vi "Parse XML.vi"(10 "Sender Host":string, 11 "Message XML String":string) -> (3 "Message":T2)   [LabVIEW 2014, in "AMC.lvlib"]
uses:
  AMC.lvlib
  Keyed Array/KeyedArray.ctl
  Keyed Array/Tools_KeyedArray.lvlib
  TypeDefs/Message.ctl
panel:
  out "Attributes":string
  out "Attributes":T1
  out "No Attributes":bool
  out "tag":string
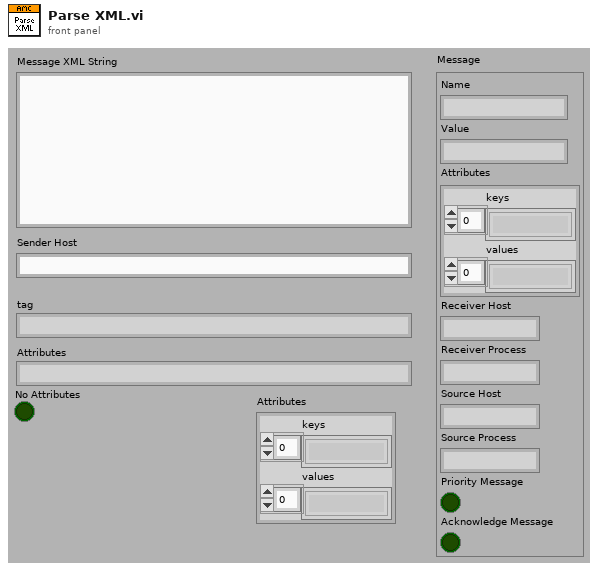
[diagram p1: front panel]
types:
  T1 = typedef "Tools_KeyedArray.lvlib/KeyedArray.ctl" = cluster{"keys":string[], "values":string[]}
  T2 = typedef "AMC.lvlib/Message.ctl" = cluster{"Name":string, "Value":string, "Attributes":T1, "Receiver Host":string, "Receiver Process":string, "Source Host":string, "Source Process":string, "Priority Message":bool, "Acknowledge Message":bool}
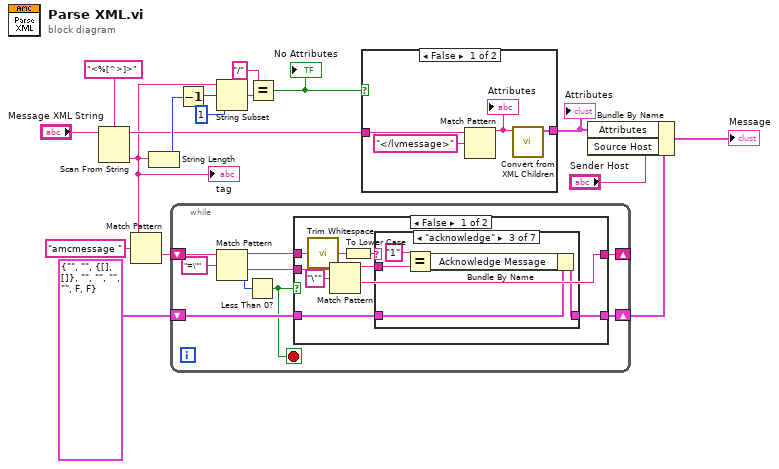
[diagram p0: block diagram]
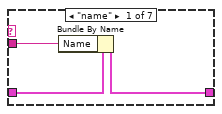
[diagram p2: hidden frame]
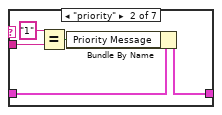
[diagram p3: hidden frame]
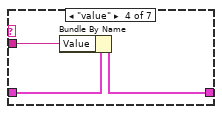
[diagram p4: hidden frame]
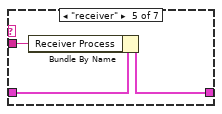
[diagram p5: hidden frame]
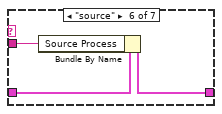
[diagram p6: hidden frame]
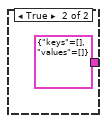
[diagram p9: hidden frame]
diagram:
  n1 = Scan From String(format string="<%[^>]>", input string="Message XML String") -> (remaining string=w9:string, output 1=w7:string)  [unwired: 2 in, 3 out]
  "tag" <- w7
  n2 = Match Pattern(string=w7, regular expression="amcmessage ") -> (after substring=w5:string)  [unwired: 4 out]
  n3 = String Length(string=w7) -> (length=w14:i32)
  n4 = while {
    shift-right: [w20] -> w3
    shift-left: T2 {"Name"="", "Value"="", "Attributes"={"keys"=[], "values"=[]}, "Receiver Host"="", "Receiver Process"="", "Source Host"="", "Source Process"="", "Priority Message"=FALSE, "Acknowledge Message"=FALSE} ("Message") -> [w21]
    shift-right: [w18] -> _
    shift-left: w5 -> [w26]
    stop <- w19 stop-if-true
    n5 = Match Pattern(string=w26, regular expression="=\"") -> (before substring=w23:string, after substring=w22:string, offset past match=w24:i32)  [unwired: 2 out]
    n6 = Less Than 0?(x=w24) -> (x < 0?=w19:bool)
    n7 = case shown="False" w19 {
      tunnel: w23 -> [w35 _]
      tunnel: w22 -> [w34 w59]
      tunnel: w21 -> [w30 w60]
      tunnel: [w29 w60] -> w20
      tunnel: [w28 w59] -> w18
      frame False {
        n8 = call <vilib>:"Trim Whitespace.vi"("string"=w35) -> ("trimmed string"=w32:string)  [unwired: 1 in]
        n9 = Match Pattern(string=w34, regular expression="\"") -> (before substring=w31:string, after substring=w28:string)  [unwired: 3 out]
        n10 = To Lower Case(string=w32) -> (all lower case string=w27:string)
        n11 = case shown="\"acknowledge\"" w27 {
          tunnel: w31 -> [w37 w42 w47 w50 w53 w56 _]
          tunnel: w30 -> [w38 w43 w48 w51 w54 w57 w58]
          tunnel: [w36 w41 w46 w49 w52 w55 w58] -> w29
          frame "name" {
            n12 = Bundle By Name(cluster=w38, "Name"=w37) -> (w36:T2)
          }
          frame "priority" {
            n13 = Equal?(x="1", y=w42) -> (x = y?=w40:bool)
            n14 = Bundle By Name(cluster=w43, "Priority Message"=w40) -> (w41:T2)
          }
          frame "acknowledge" {
            n15 = Equal?(x="1", y=w47) -> (x = y?=w45:bool)
            n16 = Bundle By Name(cluster=w48, "Acknowledge Message"=w45) -> (w46:T2)
          }
          frame "value" {
            n17 = Bundle By Name(cluster=w51, "Value"=w50) -> (w49:T2)
          }
          frame "receiver" {
            n18 = Bundle By Name(cluster=w54, "Receiver Process"=w53) -> (w52:T2)
          }
          frame "source" {
            n19 = Bundle By Name(cluster=w57, "Source Process"=w56) -> (w55:T2)
          }
          frame Default {
          }
        }
      }
      frame True {
      }
    }
  }
  n20 = Decrement(x=w14) -> (x-1=w15:i32)
  n21 = String Subset(string=w7, offset (0)=w15, length (rest)=1 ("length (rest)")) -> (substring=w12:string)
  n22 = Equal?(x="/", y=w12) -> (x = y?=w10:bool)
  "No Attributes" <- w10
  n23 = case shown="False" w10 {
    tunnel: w9 -> [w64 _]
    tunnel: [w62 T1 {"keys"=[], "values"=[]} ("keyed array")] -> w8
    frame False {
      n24 = Match Pattern(string=w64, regular expression="</lvmessage>" ("format string")) -> (before substring=w61:string)  [unwired: 4 out]
      "Attributes" <- w61
      n25 = call "Convert from XML Children.vi"("KA String"=w61) -> ("keyed array"=w62:T1)  [unwired: 1 in, 9 out]
    }
    frame True {
    }
  }
  "Attributes" <- w8
  n26 = Bundle By Name(cluster=w3, "Attributes"=w8, "Source Host"="Sender Host") -> (→"Message":T2)
